vi "TelegramBotSimpleExample.vi"() -> ()   [LabVIEW 2015]
uses:
  Telegram/Methods/TypeDefs/ReplyKeyboardMarkup.ctl
  Telegram/Methods/TypeDefs/SendMessageType.ctl
panel:
  in  "stop":bool
  out "Message":string
  out "LED":bool
  out "ConnectionStatus":bool
  # "Telegram Bot Simple Example"
  # "Default Bot name: @ATISIndBot\n\nCommand list:\n/newkbrd - create new keyboard.\nred, green, orange - keyboard buttons to changing LED clolor.\ndelete - button to delete keyboard."
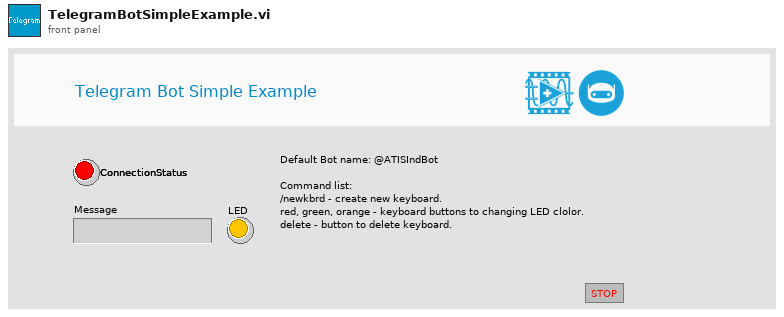
[diagram p1: front panel]
types:
  T1 = typedef "SendMessageType.ctl" = enum16{"Text", "ReplyKeyboardMarkup", "ReplyKeyboardRemove"}
  T2 = typedef "UpdateUniversal.ctl" = cluster{"update_id":u32, "message":cluster{"message_id":u32, "from":cluster{"id":u32, "first_name":string}, "chat":cluster{"id":i32, "first_name":string, "type":string}, "date":u32, "text":string, "reply_to_message":cluster{"message_id":u32, "from":cluster{"id":u32, "first_name":string}, "chat":cluster{"id":i32, "first_name":string, "type":string}, "date":u32, "text":string}}}[]
  T3 = typedef "Message.ctl" = cluster{"update_id":u32, "from":string, "text":string, "date":timestamp, "chat_id":i32, "type":string, "reply_to_message.text":string, "message_id":u32}
  T4 = typedef "ReplyKeyboardMarkup.ctl" = cluster{"keyboard":cluster{"text":string, "req_loc":bool}[][], "resize_keyboard":bool, "one_time_keyboard":bool, "selective":bool}
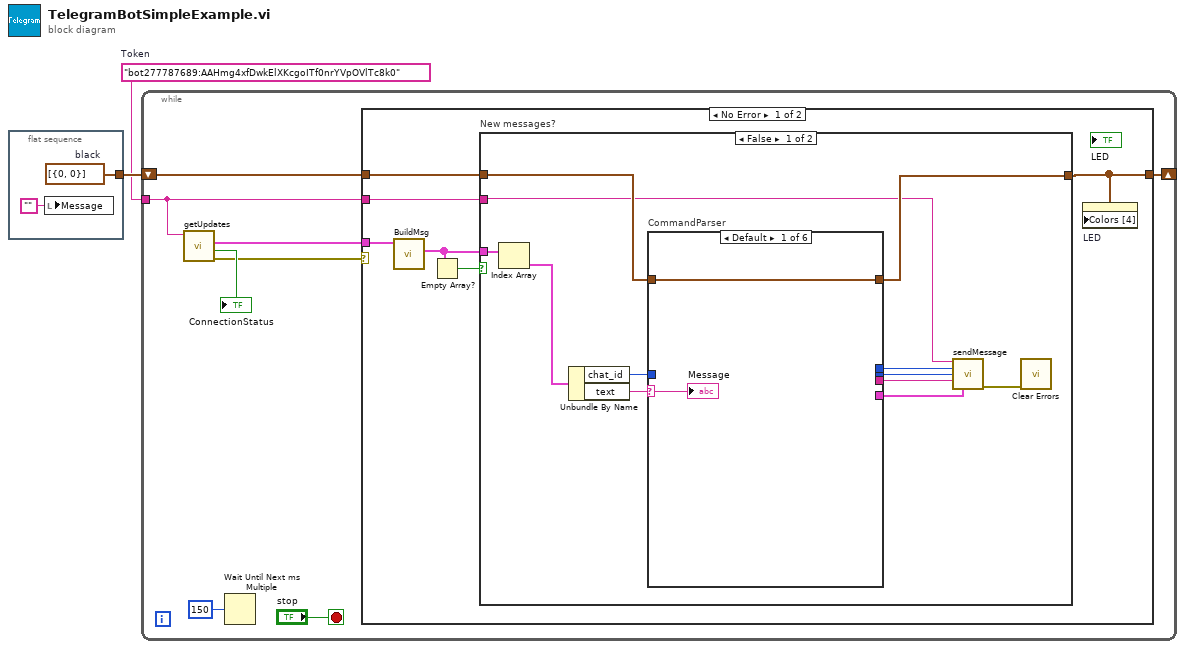
[diagram p0: block diagram]
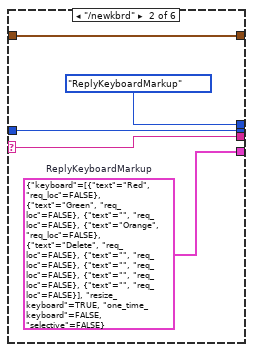
[diagram p2: hidden frame]
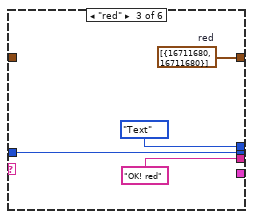
[diagram p3: hidden frame]
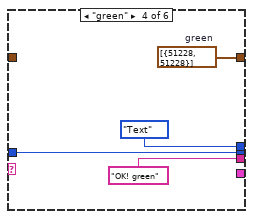
[diagram p4: hidden frame]
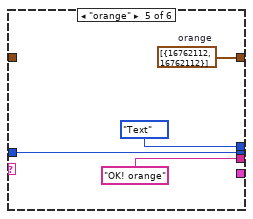
[diagram p5: hidden frame]
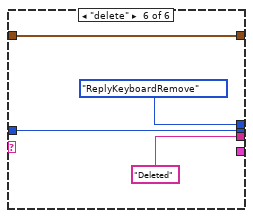
[diagram p6: hidden frame]
diagram:
  w1 = "bot277787689:AAHmg4xfDwkElXKcgoITf0nrYVpOVlTc8k0"  # Token
  n1 = flat-sequence {
    tunnel: [w4] -> w2
    frame #0 {
      w4 = cluster{u32, u32}[] [{0, 0}]  # black
      n2 = local write "Message"("") -> ()
    }
  }
  n3 = while {
    tunnel: w1 -> [w9]
    shift-right: [w6] -> _
    shift-left: w2 -> [w11]
    stop <- "stop" stop-if-true
    n4 = call "getUpdates.vi"("Token"=w9) -> ("error out"=w5:errorcluster, "ConnectionStatus"=→"ConnectionStatus":bool, "UpdateUniversal"=w7:T2)  [unwired: 7 in, 1 out]
    n5 = Wait Until Next ms Multiple(millisecond multiple=u32 150) -> ()  [unwired: 1 out]
    n6 = case shown="No Error" w5 {
      tunnel: w11 -> [w18 w55]
      tunnel: w9 -> [w17 _]
      tunnel: w7 -> [w16 _]
      tunnel: [w14 w55] -> w6
      frame No Error {
        n7 = call "BuildMsg.vi"("Result"=w16) -> ("Messages"=w15:T3[])  [unwired: 9 in, 1 out]
        n8 = Empty Array?(array=w15) -> (empty?=w13:bool)
        n9 = case "New messages?" shown="False" w13 {
          tunnel: w15 -> [w30 _]
          tunnel: w17 -> [w24 _]
          tunnel: w18 -> [w26 w54]
          tunnel: [w25 w54] -> w14
          frame False {
            n10 = Index Array(array=w30) -> (element=w29:T3)  [unwired: 1 in]
            n11 = Unbundle By Name(w29) -> ("chat_id"=w27:i32, "text"=w28:string)
            n12 = case "CommandParser" shown="Default" w28 {
              selector: w28 -> [w32 w35 _ _ _ _]
              tunnel: [_ w37 w40 w44 w48 w53] -> w21
              tunnel: w27 -> [_ w37 w40 w44 w48 w53]
              tunnel: [_ SendMessageType."ReplyKeyboardMarkup" ("MsgType") SendMessageType."Text" ("MsgType") SendMessageType."Text" ("MsgType") SendMessageType."Text" ("MsgType") SendMessageType."ReplyKeyboardRemove" ("MsgType")] -> w20
              tunnel: [_ w35 "OK! red" "OK! green" "OK! orange" "Deleted"] -> w22
              tunnel: [_ w34 _ _ _ _] -> w23
              tunnel: w26 -> [w31 w33 _ _ _ w51]
              tunnel: [w31 w33 w41 w45 w49 w51] -> w25
              frame Default {
                "Message" <- w32
              }
              frame "/newkbrd" {
                w34 = T4 {"keyboard"=[[{"text"="Red", "req_loc"=FALSE}, {"text"="Green", "req_loc"=FALSE}, {"text"="", "req_loc"=FALSE}], [{"text"="Orange", "req_loc"=FALSE}, {"text"="Delete", "req_loc"=FALSE}, {"text"="", "req_loc"=FALSE}], [{"text"="", "req_loc"=FALSE}, {"text"="", "req_loc"=FALSE}, {"text"="", "req_loc"=FALSE}]], "resize_keyboard"=TRUE, "one_time_keyboard"=FALSE, "selective"=FALSE}  # ReplyKeyboardMarkup
              }
              frame "red" {
                w41 = cluster{u32, u32}[] [{16711680, 16711680}]  # red
              }
              frame "green" {
                w45 = cluster{u32, u32}[] [{51228, 51228}]  # green
              }
              frame "orange" {
                w49 = cluster{u32, u32}[] [{16762112, 16762112}]  # orange
              }
              frame "delete" {
              }
            }
            n13 = call "sendMessage.vi"("Token"=w24, "MsgType"=w20, "ChatId"=w21, "Text"=w22, "ReplyKeyboardMarkup"=w23) -> ("error out"=w19:errorcluster)  [unwired: 10 in]
            n14 = call <vilib>:"Clear Errors.vi"("error in (no error)"=w19) -> ()  [unwired: 5 in, 2 out]
          }
          frame True {
          }
        }
        n15 = property on="LED" class="Bool (strict)"("Colors [4]"=w14) -> ()  [unwired: 2 in, 2 out]
      }
      frame Error {
      }
    }
  }
